vi "参数导入.vi"(11 "新载入系统参数路径":path) -> (1 "表首行":string[](array[string]), 2 "系统参数输出":string[][](array[string]), 3 "字符串格式输出":string)   [LabVIEW 2021]
uses:
  <vilib>/Utility/NIReport.llb/Report Type.ctl
  <vilib>/addons/_office/excel.llb/Excel Get Data ([str]).vi
  <vilib>/Utility/NIReport.llb/NI_report.lvclass
  <vilib>/Utility/NIReport.llb/NI_ReportGenerationCore.lvlib
  <vilib>/addons/_office/NI_ReportGenerationToolkit.lvlib
  <vilib>/Utility/NIReport.llb/Excel/NI_Excel.lvclass
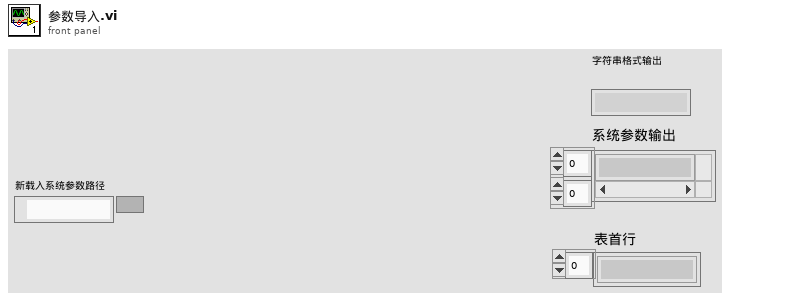
[diagram p1: front panel]
types:
  T1 = typedef "NI_ReportGenerationCore.lvlib/Report Type.ctl" = enum16{"HTML", "Word", "Excel"}
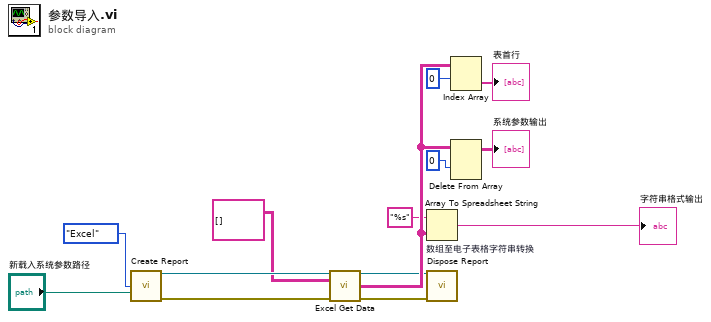
[diagram p0: block diagram]
diagram:
  n1 = call <vilib>:"Create Report.vi"("report type"=Report_Type."Excel", "template (empty)"="新载入系统参数路径") -> ("report out"=w6:refnum<class "NI_report.lvclass">, "error out"=w1:errorcluster)  [unwired: 12 in]
  n2 = call-poly <vilib>:"Excel Get Data.vi"("report in"=w6, "data type"=string[][] [], "error in (no error)"=w1) -> ("report out"=w3:refnum<class "NI_report.lvclass">, "data"=w10:string[][], "error out"=w2:errorcluster)  [unwired: 10 in]
  n3 = Array To Spreadsheet String "数组至电子表格字符串转换"(array=w10, 3:"%s" ("格式字符串")) -> (spreadsheet string=→"字符串格式输出":string)  [unwired: 1 in]
  n4 = call-dynamic "Dispose Report.vi"("report in"=w3, "error in (no error)"=w2) -> ()  [unwired: 13 in, 1 out]
  n5 = Index Array(array=w10, index (row)=0 ("索引 (行)")) -> (element=→"表首行":string[])  [unwired: 1 in]
  n6 = Delete From Array(array=w10, index (row)=0 ("索引 (行)")) -> (array with subset deleted=→"系统参数输出":string[][])  [unwired: 2 in, 1 out]
